vi "Write Variable Header (Bytes).vi"(10 "Variable Header (Bytes)":u8[](array[numeric]) format="%08b", 11 "ControlPacket in":refnum<class "ControlPacket.lvclass">) -> (3 "ControlPacket out":refnum<class "ControlPacket.lvclass">)   [LabVIEW 2013, in "ControlPacket.lvclass"]
uses:
  ControlPacket.lvclass
  ControlPacket.lvclass/ControlPacket.ctl
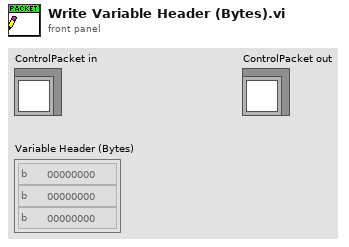
[diagram p1: front panel]
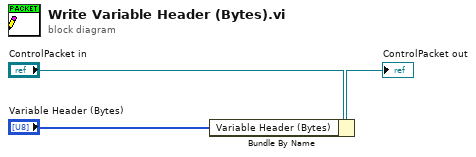
[diagram p0: block diagram]
diagram:
  n1 = Bundle By Name(cluster="ControlPacket in", "Variable Header (Bytes)"="Variable Header (Bytes)") -> (→"ControlPacket out":refnum<class "ControlPacket.lvclass">)
